vi "Utility Firmware Info.vi"(5 "Retry Attempts (0)":i32 min=0, 8 "error in":errorcluster, 11 "VISA resource name":refnum<visa-resource-name>) -> (0 "error out":errorcluster, 2 "Firmware Version":dbl, 3 "VISA resource name out":refnum<visa-resource-name>)   [LabVIEW 2020, in "ChromTech Series III Pump.lvlib"]
doc: "Returns the firmware version and part number."
uses:
  <instrlib>/ChromTech Series III Pump/ChromTech Series III Pump.lvlib
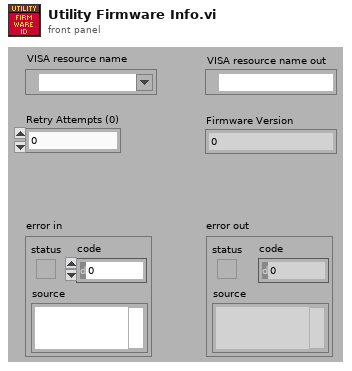
[diagram p1: front panel]
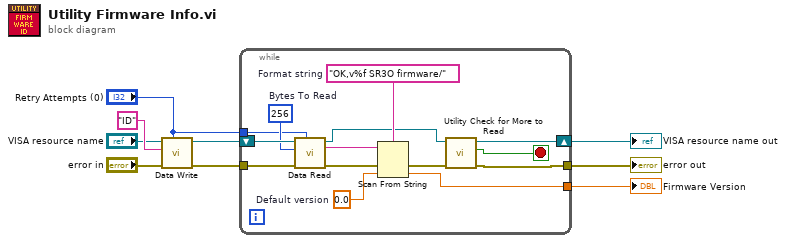
[diagram p0: block diagram]
diagram:
  n1 = call <instrlib>:"Data Write.vi"("Retry Attempts (0)"="Retry Attempts (0)", "error in (no error)"="error in", "Command"="ID", "VISA Refnum in"="VISA resource name") -> ("error out"=w6:errorcluster, "VISA Refnum out"=w5:refnum<visa-resource-name>)  [unwired: 6 in]
  n2 = while {
    tunnel: [w22] -> w8
    tunnel: "Retry Attempts (0)" -> [w14]
    shift-right: [w11] -> w2
    shift-left: w5 -> [w17]
    tunnel: w6 -> [w18]
    tunnel: [w13] -> w7
    stop <- w10 stop-if-true
    w16 = u32 256  # Bytes To Read
    w19 = 0.0  # Default version
    w23 = "OK,v%f SR3O firmware/"  # Format string
    n3 = call <instrlib>:"Data Read.vi"("Retry Attempts (0)"=w14, "error in (no error)"=w18, "Bytes to read"=w16, "VISA Refnum in"=w17) -> ("error out"=w21:errorcluster, "read buffer"=w15:string, "VISA Refnum out"=w12:refnum<visa-resource-name>)  [unwired: 5 in]
    n4 = Scan From String(format string=w23, input string=w15, error in=w21, default 1=w19) -> (error out=w20:errorcluster, output 1=w22:dbl)  [unwired: 1 in, 2 out]
    n5 = call <instrlib>:"Utility Check for More to Read.vi"("error in (no error)"=w20, "VISA Refnum in"=w12) -> ("error out (unchanged)"=w13:errorcluster, "More to read?"=w10:bool, "VISA Refnum out"=w11:refnum<visa-resource-name>)  [unwired: 7 in]
  }
  "VISA resource name out" <- w2
  "error out" <- w7
  "Firmware Version" <- w8
